vi "setValvesArduinosSinglePuffNew.vi"(8 "milliseconds to wait":u32=100, 10 "valve data close":bool[](array[boolean])=[FALSE, FALSE, FALSE, FALSE, FALSE, FALSE, FALSE, FALSE], 11 "valve data open":bool[](array[boolean])=[FALSE, FALSE, FALSE, FALSE, FALSE, FALSE, FALSE, FALSE]) -> ()   [LabVIEW 2012]
uses:
  GlobalValves.vi
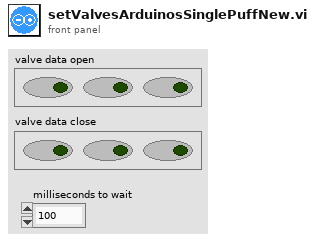
[diagram p1: front panel]
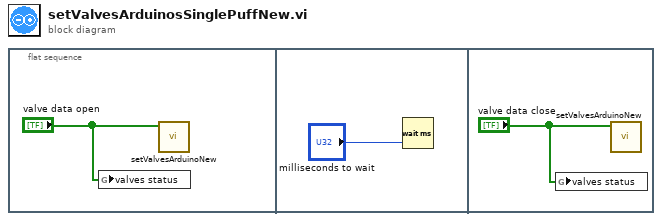
[diagram p0: block diagram]
diagram:
  n1 = flat-sequence {
    frame #0 {
      n2 = global write "GlobalValves.vi" "valves status"("valve data open") -> ()
      n3 = call "setValvesArduinoNew.vi"("valve data"="valve data open") -> ()  [unwired: 11 in]
    }
    frame #1 {
      n4 = Wait (ms)(milliseconds to wait="milliseconds to wait") -> ()  [unwired: 1 out]
    }
    frame #2 {
      n5 = global write "GlobalValves.vi" "valves status"("valve data close") -> ()
      n6 = call "setValvesArduinoNew.vi"("valve data"="valve data close") -> ()  [unwired: 11 in]
    }
  }
